vi "Digital Tach Timing Ex.vi"(5 "reset? (True)":bool=TRUE, 9 "counter task type":enum16{"period measurement", "event counting"}(ring)=enum."event counting", 10 "counter timebase [Hz]":dbl=20000000.0 format="%.0p", 11 "tach counts":u32[](array[numeric])) -> (1 "number of pulses":i32, 3 "pulse positions [s]":dbl[](array[numeric]) format="%.2f")   [LabVIEW 2017, in "SoundVib_TachProcess.lvlib"]
doc: "Times the tachometer signal acquired by a digital counter."
uses:
  <vilib>/addons/Sound and Vibration/Order Analysis/Tach Process/SoundVib_TachProcess.lvlib
panel:
  # "Digital Tach Timing"
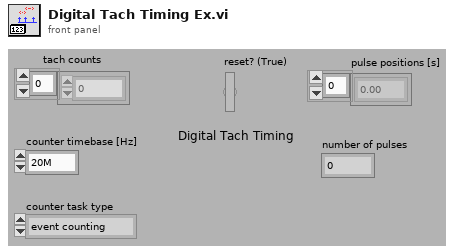
[diagram p1: front panel]
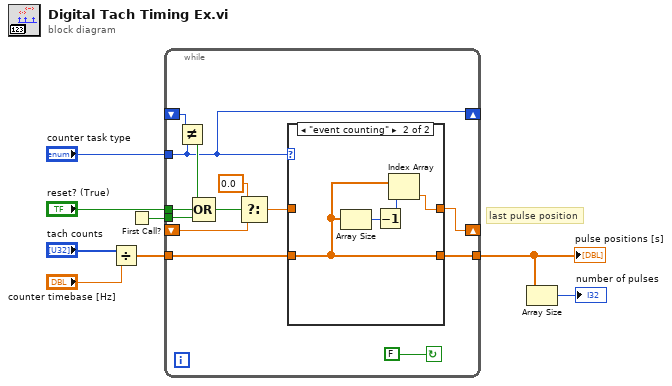
[diagram p0: block diagram]
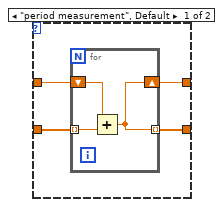
[diagram p2: hidden frame]
diagram:
  # "last pulse position"
  n1 = Divide(x="tach counts", y="counter timebase [Hz]") -> (x/y=w4:dbl[])
  n2 = First Call?() -> (First Call?: T/F=w2:bool)
  n3 = while {
    tunnel: "counter task type" -> [w16]
    tunnel: w4 -> [w14]
    tunnel: "reset? (True)" -> [w19]
    shift-right: [w16] -> _
    shift-left: _ -> [w20]
    tunnel: w2 -> [w17]
    tunnel: [w9] -> w1
    shift-right: [w15] -> _
    shift-left: _ -> [w10]
    stop <- FALSE continue-if-true
    n4 = Not Equal?(x=w20, y=w16) -> (x != y?=w18:bool)
    n5 = Compound Arithmetic op=OR(w18, w19, w17) -> (w11:bool)
    n6 = Select(t=0.0, s=w11, f=w10) -> (s? t:f=w12:dbl)
    n7 = case shown="\"event counting\"" w16 {
      tunnel: [w24 w32] -> w9
      tunnel: [w23 w29] -> w15
      tunnel: w14 -> [w25 w32]
      tunnel: w12 -> [w22 _]
      frame "period measurement", Default {
        n8 = for {
          shift-right: [w27] -> w23
          shift-left: w22 -> [w28]
          tunnel: [w27] -> w24 mode=indexing
          tunnel: w25 -> [w26] mode=indexing
          n9 = Add(x=w28, y=w26) -> (x+y=w27:dbl)
        }
      }
      frame "event counting" {
        n10 = Array Size(array=w32) -> (size(s)=w31:i32)
        n11 = Decrement(x=w31) -> (x-1=w30:i32)
        n12 = Index Array(array=w32, index=w30) -> (element=w29:dbl)
      }
    }
  }
  "pulse positions [s]" <- w1
  n13 = Array Size(array=w1) -> (size(s)=→"number of pulses":i32)
